vi "Check Action.vi"(6 "HRS Time":dbl, 7 "Values In":dbl[](array[numeric]), 8 "error in (no error)":errorcluster, 11 "LatchedValve in":refnum<class "LatchedValve.lvclass">) -> (0 "error out":errorcluster, 1 "Do Action":bool, 2 "Action":T1, 3 "LatchedValve out":refnum<class "LatchedValve.lvclass">, 5 "Values":dbl[](array[numeric]))   [LabVIEW 2020, in "VolatusControl.lvlib" / "LatchedValve.lvclass"]
uses:
  LatchedValve.lvclass
  Valve Action.ctl
  Volatus/MessageQ/MessageQ.lvclass
  LatchedValve.lvclass/LatchedValve.ctl
  State.ctl
  VolatusControl.lvlib
  lv-vecto/Vecto/Vecto.lvlib
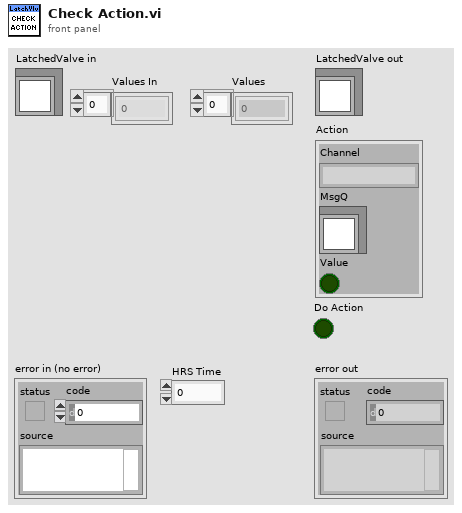
[diagram p1: front panel]
types:
  T1 = typedef "VolatusControl.lvlib/Valve Action.ctl" = cluster{"Channel":string, "MsgQ":refnum<class "MessageQ.lvclass">, "Value":bool}
  T2 = typedef "VolatusControl.lvlib/LatchedValve.lvclass/State.ctl" = enum16{"Idle", "Cmd Dir", "Settle Dir", "Actuate", "Deactivate"}
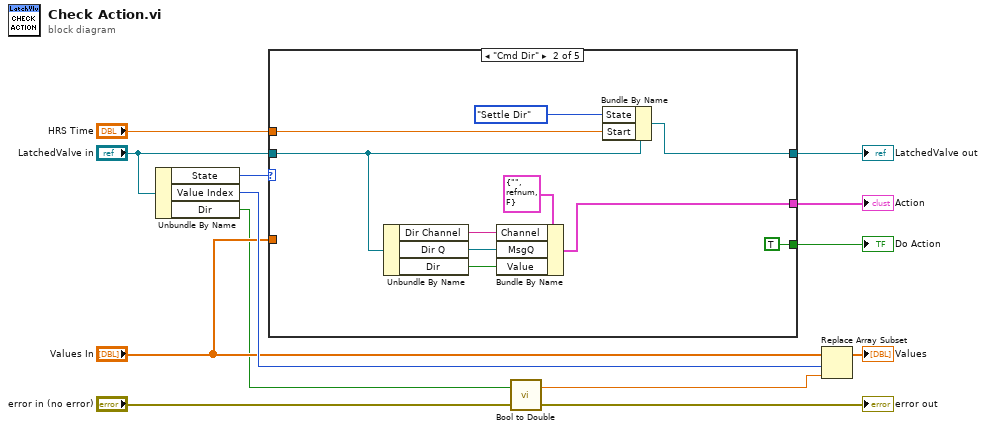
[diagram p0: block diagram]
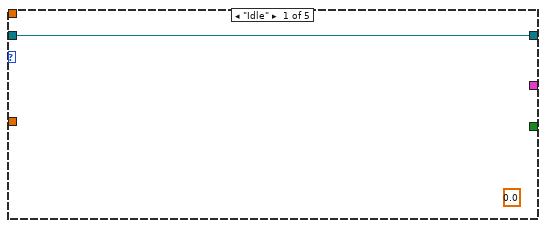
[diagram p2: hidden frame]
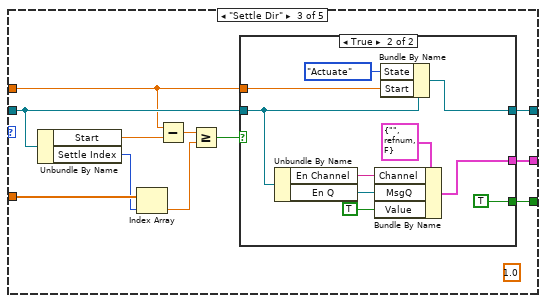
[diagram p3: hidden frame]
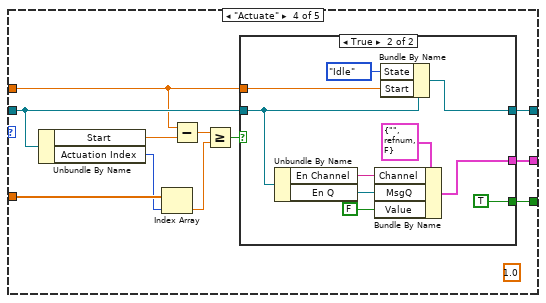
[diagram p5: hidden frame]
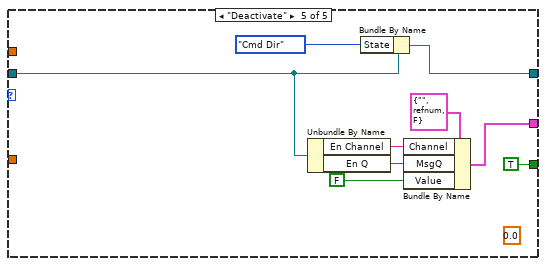
[diagram p7: hidden frame]
diagram:
  n1 = Unbundle By Name("LatchedValve in") -> ("State"=w11:T2, "Value Index"=w4:i32, "Dir"=w1:bool)
  n2 = case shown="\"Cmd Dir\"" w11 {
    tunnel: "LatchedValve in" -> [w13 w19 w31 w53 w69]
    tunnel: [w13 w17 w32 w54 w75] -> w10
    tunnel: [_ w22 w34 w56 w70] -> w9
    tunnel: [_ TRUE w27 w49 TRUE] -> w5
    tunnel: "HRS Time" -> [_ w16 w30 w52 _]
    tunnel: "Values In" -> [_ _ w26 w48 _]
    frame "Idle" {
      (unwired) 0.0
    }
    frame "Cmd Dir" {
      n3 = Unbundle By Name(w19) -> ("Dir Channel"=w20:string, "Dir Q"=w21:refnum<class "MessageQ.lvclass">, "Dir"=w14:bool)
      n4 = Bundle By Name(cluster=T1 {"Channel"="", "MsgQ"=refnum, "Value"=FALSE} ("Action"), "Channel"=w20, "MsgQ"=w21, "Value"=w14) -> (w22:T1)
      n5 = Bundle By Name(cluster=w19, "State"=State."Settle Dir", "Start"=w16) -> (w17:refnum<class "LatchedValve.lvclass">)
    }
    frame "Settle Dir" {
      (unwired) 1.0
      n6 = Unbundle By Name(w31) -> ("Start"=w33:dbl, "Settle Index"=w25:i32)
      n7 = Index Array(array=w26, index=w25) -> (element=w24:dbl)
      n8 = Subtract(x=w30, y=w33) -> (x-y=w29:dbl)
      n9 = Greater Or Equal?(x=w29, y=w24) -> (x >= y?=w28:bool)
      n10 = case shown="True" w28 {
        tunnel: [_ w44] -> w34
        tunnel: [w35 w40] -> w32
        tunnel: w31 -> [w35 w39]
        tunnel: w30 -> [_ w37]
        tunnel: [_ TRUE] -> w27
        frame False {
        }
        frame True {
          n11 = Unbundle By Name(w39) -> ("En Channel"=w42:string, "En Q"=w41:refnum<class "MessageQ.lvclass">)
          n12 = Bundle By Name(cluster=T1 {"Channel"="", "MsgQ"=refnum, "Value"=FALSE} ("Action"), "Channel"=w42, "MsgQ"=w41, "Value"=TRUE) -> (w44:T1)
          n13 = Bundle By Name(cluster=w39, "State"=State."Actuate", "Start"=w37) -> (w40:refnum<class "LatchedValve.lvclass">)
        }
      }
    }
    frame "Actuate" {
      (unwired) 1.0
      n14 = Unbundle By Name(w53) -> ("Start"=w55:dbl, "Actuation Index"=w47:i32)
      n15 = Index Array(array=w48, index=w47) -> (element=w46:dbl)
      n16 = Subtract(x=w52, y=w55) -> (x-y=w51:dbl)
      n17 = Greater Or Equal?(x=w51, y=w46) -> (x >= y?=w50:bool)
      n18 = case shown="True" w50 {
        tunnel: [_ w66] -> w56
        tunnel: [w57 w62] -> w54
        tunnel: w53 -> [w57 w61]
        tunnel: w52 -> [_ w59]
        tunnel: [_ TRUE] -> w49
        frame False {
        }
        frame True {
          n19 = Unbundle By Name(w61) -> ("En Channel"=w64:string, "En Q"=w63:refnum<class "MessageQ.lvclass">)
          n20 = Bundle By Name(cluster=T1 {"Channel"="", "MsgQ"=refnum, "Value"=FALSE} ("Action"), "Channel"=w64, "MsgQ"=w63, "Value"=FALSE) -> (w66:T1)
          n21 = Bundle By Name(cluster=w61, "State"=State."Idle", "Start"=w59) -> (w62:refnum<class "LatchedValve.lvclass">)
        }
      }
    }
    frame "Deactivate" {
      (unwired) 0.0
      n22 = Unbundle By Name(w69) -> ("En Channel"=w71:string, "En Q"=w72:refnum<class "MessageQ.lvclass">)
      n23 = Bundle By Name(cluster=w69, "State"=State."Cmd Dir") -> (w75:refnum<class "LatchedValve.lvclass">)
      n24 = Bundle By Name(cluster=T1 {"Channel"="", "MsgQ"=refnum, "Value"=FALSE} ("Action"), "Channel"=w71, "MsgQ"=w72, "Value"=FALSE) -> (w70:T1)
    }
  }
  "LatchedValve out" <- w10
  "Action" <- w9
  "Do Action" <- w5
  n25 = call "Bool to Double.vi"("Bool"=w1) -> ("Double"=w2:dbl)  [unwired: 2 in]
  n26 = Replace Array Subset(array="Values In", new element=w2, index=w4) -> (→"Values":dbl[])
  "error out" <- "error in (no error)"
